vi "Teleop.vi"(10 "Match Info":T1={"Autonomous Elapsed Seconds"=0.0, "TeleOp Elapsed Seconds"=0.0, "Disabled Elapsed Seconds"=0.0, "Visited Autonomous"=FALSE, "Visited TeleOp"=FALSE, "Visited Disabled"=FALSE, "Autonomous Settings"={"Autonomous Style"=enum."Independent", "VI Refnum"=refnum}}, 11 "Call Context":T2) -> ()   [LabVIEW 2018]
doc: "This VI is called for each enabled TeleOp packet received from the DS. It is typically used to read from joysticks and other inputs and update I/O or setpoints for timed control loops. It should complete and return within 20 milliseconds or risk missing DS packets."
uses:
  <vilib>/Rock Robotics/WPI/DriverStation/WPI_DriverStationDerivedRobotMode.ctl
  <vilib>/Rock Robotics/WPI/DriverStation/WPI_DriverStationMatch Info.ctl
  <vilib>/Rock Robotics/WPI/Utilities/WPI_GetSetVariantRefNum.vi
  <vilib>/Rock Robotics/WPI/RobotDrive/WPI_RobotDriveMecanumDrive_Cartesian.vi
  <vilib>/Rock Robotics/WPI/RobotDrive/WPI_RobotDriveArcadeDrive_Standard(NoSaturation).vi
  <vilib>/Rock Robotics/WPI/Solenoid/WPI_SolenoidValue.ctl
  <vilib>/Rock Robotics/WPI/Solenoid/WPI_SolenoidSetEnum.vi
panel:
  out "Distance":dbl
  out "Magnet sensed 2":bool
  out "Magnet sensed 1":bool
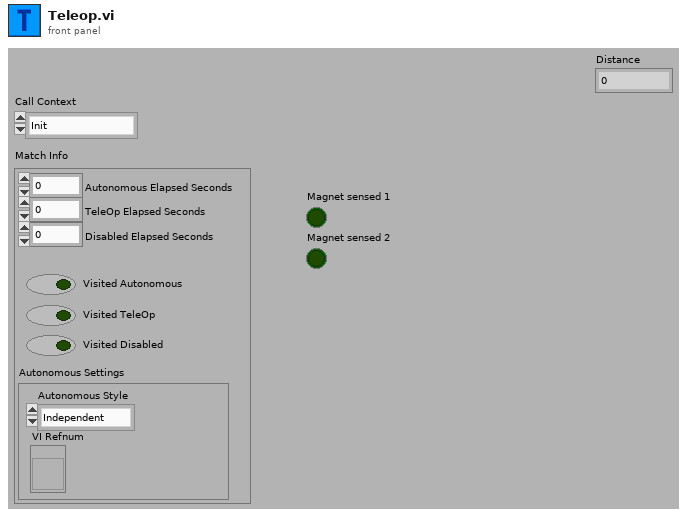
[diagram p1: front panel]
types:
  T1 = typedef "WPI_DriverStationMatch Info.ctl" = cluster{"Autonomous Elapsed Seconds":dbl, "TeleOp Elapsed Seconds":dbl, "Disabled Elapsed Seconds":dbl, "Visited Autonomous":bool, "Visited TeleOp":bool, "Visited Disabled":bool, "Autonomous Settings":cluster{"Autonomous Style":enum16{"Iterative", "Independent"}, "VI Refnum":refnum<vi>}}
  T2 = typedef "WPI_DriverStationDerivedRobotMode.ctl" = enum16{"Init", "Execute", "Stop"}
  T3 = typedef "WPI_JoystickDevRef.ctl" = cluster{"Device":T4}
  T4 = typedef "WPI_JoystickDeviceEnum.ctl" = enum16{"USB 0", "USB 1", "USB 2", "USB 3", "USB 4", "USB 5"}
  T5 = typedef "WPI_EncoderDevRef.ctl" = cluster{"DevStatus":errorcluster, "EncoderIndex":T6, "CounterIndex":T7, "DistancePerCount":dbl, "Decoding Type":T8}
  T6 = typedef "FPGA_EncoderIdx.ctl" = enum8{"Enc 0", "Enc 1", "Enc 2", "Enc 3", "Enc 4", "Enc 5", "Enc 6", "Enc 7", "Invalid"}
  T7 = typedef "FPGA_CounterCtrSystemIndex.ctl" = enum8{"Ctr 0", "Ctr 1", "Ctr 2", "Ctr 3", "Ctr 4", "Ctr 5", "Ctr 6", "Ctr 7", "Invalid"}
  T8 = typedef "WPI_EncoderType.ctl" = enum16{"1x", "2x", "4x"}
  T9 = typedef "WPI_SolenoidValue.ctl" = enum16{"Off", "On", "Forward", "Reverse"}
  T10 = typedef "WPI_DigitalInputDevRef.ctl" = cluster{"DevStatus":errorcluster, "DIO Channel":T11}
  T11 = typedef "FPGA_DIOChannel.ctl" = enum8{"DIO 0", "DIO 1", "DIO 2", "DIO 3", "DIO 4", "DIO 5", "DIO 6", "DIO 7", "DIO 8", "DIO 9", "DIO MXP 0", "DIO MXP 1", "DIO MXP 2", "DIO MXP 3", "DIO MXP 4", "DIO MXP 5", "DIO MXP 6", "DIO MXP 7", "DIO MXP 8", "DIO MXP 9", "DIO MXP 10", "DIO MXP 11", "DIO MXP 12", "DIO MXP 13", "DIO MXP 14", "DIO MXP 15", "SPI Port CS1", "SPI Port CS2", "SPI Port CS3", "SPI Port MISO", "SPI Port MOSI", "Invalid"}
  T12 = typedef "WPI_SolenoidDevRef.ctl" = cluster{"DevStatus":errorcluster, "Pneumatics Control Module":u8, "Forward Solenoid Channel":T13, "Reverse Solenoid Channel":T13}
  T13 = typedef "WPI_SolenoidChannel.ctl" = enum8{"Solenoid 0", "Solenoid 1", "Solenoid 2", "Solenoid 3", "Solenoid 4", "Solenoid 5", "Solenoid 6", "Solenoid 7", "Invalid"}
  T14 = cluster{"Axes[0]":dbl, "Axes[1]":dbl, "Axes[2]":dbl, "Axes[3]":dbl, "Axes[4]":dbl, "Axes[5]":dbl, "Axes[6]":dbl, "Axes[7]":dbl, "Axes[8]":dbl}
  T15 = typedef "WPI_CompressorDevRef.ctl" = cluster{"DevStatus":errorcluster, "Pneumatics Control Module":u8}
  T16 = typedef "WPI_RobotDriveDevRef.ctl" = cluster{"DevStatus":errorcluster, "Motors[]":T17[], "Square Inputs":bool, "Max Output":dbl}
  T17 = typedef "WPI_MotorControlDeviceRef.ctl" = cluster{"DeviceStatus":errorcluster, "Type":T18, "PWM":cluster{"PWM Channel":T19, "DeadBand":T20}, "CAN":cluster{"Device Number":u8, "SetOutput VI Ref":variant, "GetOutput VI Ref":variant, "Enable VI Ref":variant, "Disable VI Ref":variant, "Data":variant}, "Invert":bool, "DIO PWM":cluster{"PWM \"Enable\" Channel":T19, "DIOChannel":T11, "PWM Rate":dbl}}
  T18 = typedef "WPI_MotorControlType.ctl" = enum16{"PWM", "CAN", "DIO PWM"}
  T19 = typedef "FPGA_DIOPWMChannel.ctl" = enum8{"PWM 0", "PWM 1", "PWM 2", "PWM 3", "PWM 4", "PWM 5", "PWM 6", "PWM 7", "PWM 8", "PWM 9", "PWM MXP 0", "PWM MXP 1", "PWM MXP 2", "PWM MXP 3", "PWM MXP 4", "PWM MXP 5", "PWM MXP 6", "PWM MXP 7", "PWM MXP 8", "PWM MXP 9", "Invalid"}
  T20 = typedef "WPI_PWMDeadband.ctl" = cluster{"Name":string, "maxPositivePwm":i32, "minPositivePwm":i32, "centerPwm":i32, "maxNegativePwm":i32, "minNegativePwm":i32, "angularRange":u16}
  T21 = cluster{"Buttons[0]":bool, "Buttons[1]":bool, "Buttons[2]":bool, "Buttons[3]":bool, "Buttons[4]":bool, "Buttons[5]":bool, "Buttons[6]":bool, "Buttons[7]":bool, "Buttons[8]":bool, "Buttons[9]":bool, "Buttons[10]":bool, "Buttons[11]":bool}
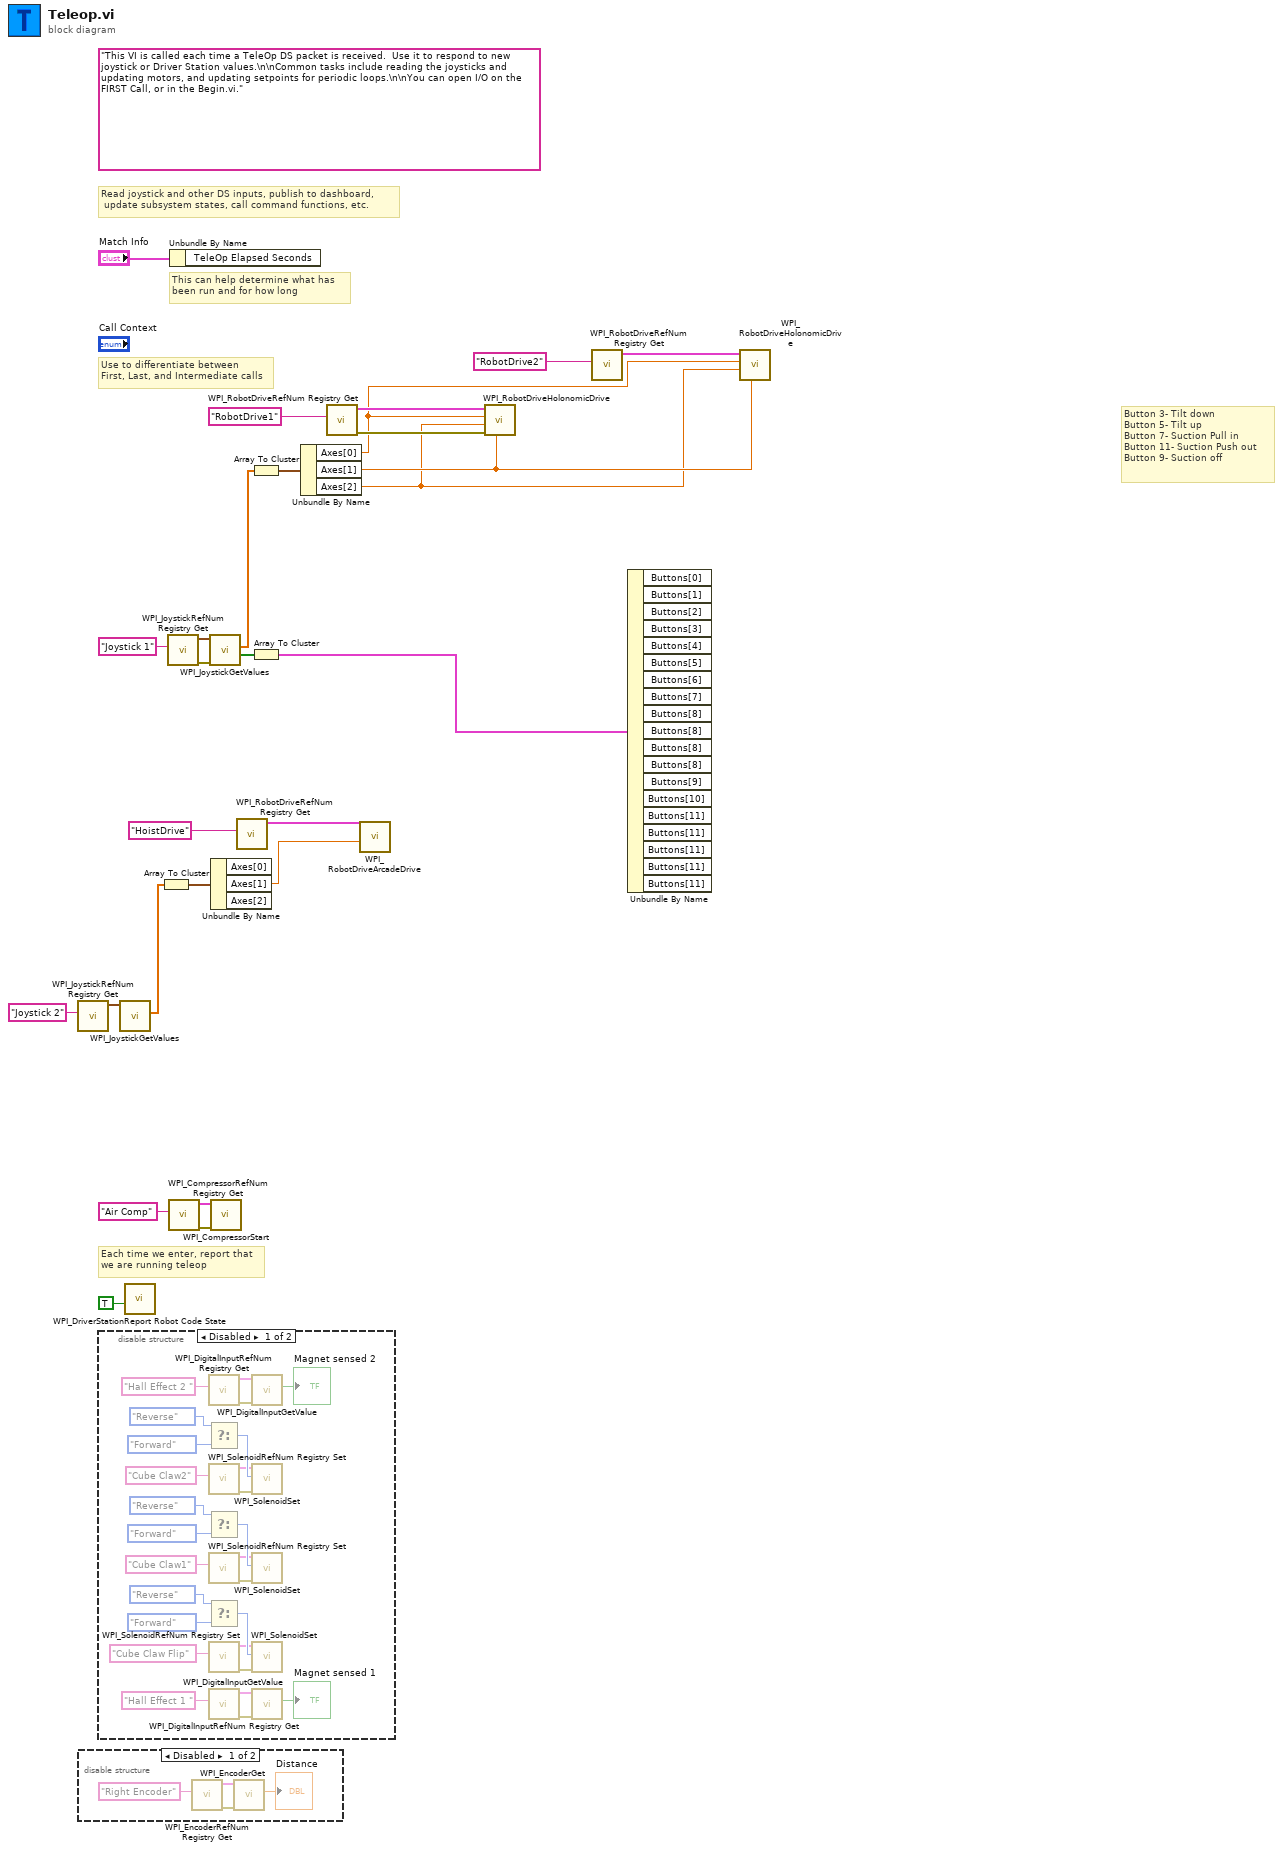
[diagram p0: block diagram]
diagram:
  (unwired) "This VI is called each time a TeleOp DS packet is received.  Use it to respond to new joystick or Driver Station values.\n\nCommon tasks include reading the joysticks and updating motors, and updating setpoints for periodic loops.\n\nYou can open I/O on the FIRST Call, or in the Begin.vi."
  # "Button 3- Tilt down\nButton 5- Tilt up\nButton 7- Suction Pull in\nButton 11- Suction Push out\nButton 9- Suction off"
  # "Read joystick and other DS inputs, publish to dashboard,\n update subsystem states, call command functions, etc."
  # "Each time we enter, report that\nwe are running teleop"
  # "Use to differentiate between\nFirst, Last, and Intermediate calls"
  # "This can help determine what has\nbeen run and for how long"
  n1 = call <vilib>:"WPI_JoystickRefNum Registry Get.vi"("refnum name"="Joystick 2") -> ("JoystickDevRef"=w6:T3)  [unwired: 9 in, 1 out]
  n2 = disable-structure shown="Disabled" {
    frame Disabled {
      n3 = call <vilib>:"WPI_EncoderRefNum Registry Get.vi"("refnum name"="Right Encoder") -> ("error out"=w30:errorcluster, "EncoderDevRef"=w31:T5)  [unwired: 9 in]
      n4 = call <vilib>:"WPI_EncoderGet.vi"("error in (no error)"=w30, "EncoderDevRef"=w31) -> ("Distance"=→"Distance":dbl)  [unwired: 4 in, 5 out]
    }
    frame Enabled {
    }
  }
  n5 = disable-structure shown="Disabled" {
    frame Disabled {
      n6 = call <vilib>:"WPI_DigitalInputRefNum Registry Get.vi"("refnum name"="Hall Effect 2 ") -> ("error out"=w39:errorcluster, "DigitalInputDevRef"=w38:T10)  [unwired: 9 in]
      n7 = Select(t=WPI_SolenoidValue."Reverse" ("Value"), f=WPI_SolenoidValue."Forward" ("Value")) -> (s? t:f=w54:T9)  [unwired: 1 in]
      n8 = call <vilib>:"WPI_SolenoidRefNum Registry Set.vi"("refnum name"="Cube Claw2") -> ("error out"=w53:errorcluster, "SolenoidDevRef"=w52:T12)  [unwired: 9 in]
      n9 = Select(t=WPI_SolenoidValue."Reverse" ("Value"), f=WPI_SolenoidValue."Forward" ("Value")) -> (s? t:f=w51:T9)  [unwired: 1 in]
      n10 = call <vilib>:"WPI_SolenoidRefNum Registry Set.vi"("refnum name"="Cube Claw1") -> ("error out"=w50:errorcluster, "SolenoidDevRef"=w49:T12)  [unwired: 9 in]
      n11 = Select(t=WPI_SolenoidValue."Reverse" ("Value"), f=WPI_SolenoidValue."Forward" ("Value")) -> (s? t:f=w57:T9)  [unwired: 1 in]
      n12 = call <vilib>:"WPI_SolenoidRefNum Registry Set.vi"("refnum name"="Cube Claw Flip") -> ("error out"=w56:errorcluster, "SolenoidDevRef"=w55:T12)  [unwired: 9 in]
      n13 = call <vilib>:"WPI_DigitalInputRefNum Registry Get.vi"("refnum name"="Hall Effect 1 ") -> ("error out"=w36:errorcluster, "DigitalInputDevRef"=w35:T10)  [unwired: 9 in]
      n14 = call <vilib>:"WPI_DigitalInputGetValue.vi"("error in (no error)"=w39, "DigitalInputDevRef"=w38) -> ("Value"=→"Magnet sensed 2":bool)  [unwired: 7 in, 2 out]
      n15 = call-poly <vilib>:"WPI_SolenoidSet.vi"("error in (no error)"=w53, "Value"=w54, "SolenoidDevRef"=w52) -> ()  [unwired: 7 in, 2 out]
      n16 = call-poly <vilib>:"WPI_SolenoidSet.vi"("error in (no error)"=w50, "Value"=w51, "SolenoidDevRef"=w49) -> ()  [unwired: 7 in, 2 out]
      n17 = call-poly <vilib>:"WPI_SolenoidSet.vi"("error in (no error)"=w56, "Value"=w57, "SolenoidDevRef"=w55) -> ()  [unwired: 7 in, 2 out]
      n18 = call <vilib>:"WPI_DigitalInputGetValue.vi"("error in (no error)"=w36, "DigitalInputDevRef"=w35) -> ("Value"=→"Magnet sensed 1":bool)  [unwired: 7 in, 2 out]
    }
    frame Enabled {
    }
  }
  n19 = call <vilib>:"WPI_JoystickGetValues.vi"("JoystickDevRef"=w6) -> ("Axes"=w3:dbl[])  [unwired: 6 in, 4 out]
  n20 = call <vilib>:"WPI_DriverStationReport Robot Code State.vi"("TeleOp"=TRUE ("Autonomous")) -> ()  [unwired: 10 in, 1 out]
  n21 = Array To Cluster(array=w3) -> (cluster=w4:T14)
  n22 = call <vilib>:"WPI_JoystickRefNum Registry Get.vi"("refnum name"="Joystick 1") -> ("error out"=w22:errorcluster, "JoystickDevRef"=w21:T3)  [unwired: 9 in]
  n23 = call <vilib>:"WPI_CompressorRefNum Registry Get.vi"("refnum name"="Air Comp") -> ("error out"=w18:errorcluster, "CompressorDevRef"=w17:T15)  [unwired: 9 in]
  n24 = Unbundle By Name("Match Info") -> ()  [unwired: 1 out]
  n25 = call <vilib>:"WPI_JoystickGetValues.vi"("error in (no error)"=w22, "JoystickDevRef"=w21) -> ("Buttons"=w16:bool[], "Axes"=w13:dbl[])  [unwired: 5 in, 3 out]
  n26 = Unbundle By Name(w4) -> ("Axes[1]"=w1:dbl)  [unwired: 2 out]
  n27 = call <vilib>:"WPI_CompressorStart.vi"("error in (no error)"=w18, "CompressorDevRef"=w17) -> ()  [unwired: 8 in, 2 out]
  n28 = call <vilib>:"WPI_RobotDriveRefNum Registry Get.vi"("refnum name"="HoistDrive") -> ("RobotDriveDevRef"=w2:T16)  [unwired: 9 in, 1 out]
  n29 = Array To Cluster(array=w13) -> (cluster=w14:T14)
  n30 = Array To Cluster(array=w16) -> (cluster=w15:T21)
  n31 = Unbundle By Name(w14) -> ("Axes[0]"=w8:dbl, "Axes[1]"=w10:dbl, "Axes[2]"=w9:dbl)
  n32 = call <vilib>:"WPI_RobotDriveRefNum Registry Get.vi"("refnum name"="RobotDrive1") -> ("error out"=w23:errorcluster, "RobotDriveDevRef"=w24:T16)  [unwired: 9 in]
  n33 = call-poly <vilib>:"WPI_RobotDriveArcadeDrive.vi"("Y axis value"=w1, "RobotDriveDevRef"=w2) -> ()  [unwired: 7 in, 3 out]
  n34 = call-poly <vilib>:"WPI_RobotDriveHolonomicDrive.vi"("Rotation"=w10, "error in (no error)"=w23, "Y"=w9, "X"=w8, "RobotDriveDevRef"=w24) -> ()  [unwired: 4 in, 3 out]
  n35 = call <vilib>:"WPI_RobotDriveRefNum Registry Get.vi"("refnum name"="RobotDrive2") -> ("RobotDriveDevRef"=w11:T16)  [unwired: 9 in, 1 out]
  n36 = Unbundle By Name(w15) -> ()  [unwired: 19 out]
  n37 = call-poly <vilib>:"WPI_RobotDriveHolonomicDrive.vi"("Rotation"=w10, "Y"=w9, "X"=w8, "RobotDriveDevRef"=w11) -> ()  [unwired: 5 in, 3 out]
